vi "Case prova.vi"(0 "control":bool) -> (1 "Numeric":i16, 2 "Led booleano":bool)   [LabVIEW 2012]
panel:
  # "Esercizio:"
  # "Se CONTROL è on: LED acceso e numeric = 1\n\nSe CONTROL è off: LED spento e numeric = 0"
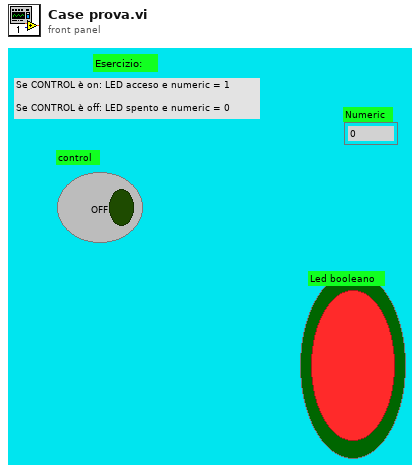
[diagram p1: front panel]
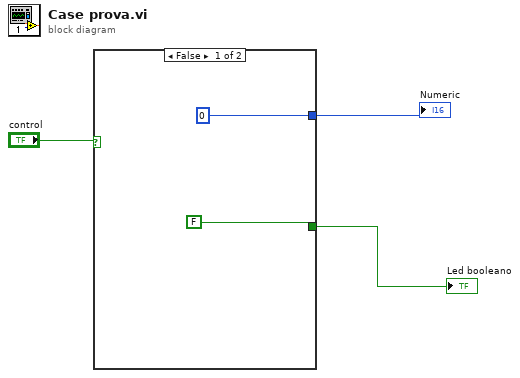
[diagram p0: block diagram]
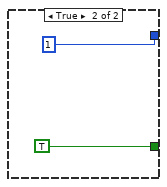
[diagram p2: hidden frame]
diagram:
  n1 = case shown="False" "control" {
    tunnel: [0 1] -> w2
    tunnel: [FALSE TRUE] -> w1
    frame False {
    }
    frame True {
    }
  }
  "Numeric" <- w2
  "Led booleano" <- w1
